vi "MAIN_STANDALONE.vi"() -> ()   [LabVIEW 2019]
uses:
  Type_defs/INPUT TEST.ctl
  Type_defs/OUTPUTS_TEST.ctl
  LVPROJ_CONFIG_ESTACION/Type_defs/Coordenadas_estacion.ctl
  LVPROJ_CREAR BANDEJAS/Type_defs/Data_Bandeja.ctl
  Type_defs/State_main.ctl
  LVPROJ_MOVIMIENTO_CABEZAL/LABVIEW_MOVIMIENTO/MOVIMIENTO CABEZAL/Typedefs/Comandos.ctl
  LVPROJ_MOVIMIENTO_CABEZAL/LABVIEW_MOVIMIENTO/MOVIMIENTO CABEZAL/Typedefs/Estados_arduino.ctl
  <vilib>/Instr/_visa.llb/VISA Configure Serial Port (Instr).vi
  <vilib>/Utility/error.llb/Error Cluster From Error Code.vi
  <vilib>/ErrorRing/Error Ring.xnode
  SHARED VI'S/SHARED VI'S.lvlib
panel:
  out "datos leídos por arduino":string
  out "CONEXION CON ARDUINO":bool
  out "read buffer 2":string
  out "read buffer":string
  out "trama datos enviada":string
  out "datos enviados = datos leídos?":bool
  out "Error Out":errorcluster
  in  "Error In":errorcluster
  in  "Tab Control":enum32{"PANEL USUARIO", "VER CONFIG ACTUAL"}(tab)
  in  "COMENZAR TEST":bool
  in  "EXIT":bool
  in  "DETENER TEST":bool
  in  "ENVIAR PARAMETROS DE TEST":bool
  in  "TEST ASICS INPUT":T1={"COORD. IN X"=0, "COORD IN Y"=0, "COORD OK X"=0, "COORD OK Y"=0, "COORD NOK X"=0, "COORD NOK Y"=0, "NºASICS A TESTEAR"=1, "SELECCIÓN DE TEST"=enum."TEST ASICS LST", "CUENTA ASICS"=0, "OPERADOR"="Javier Morales"}
  out "INDICADORES DE TEST":T2
  out "ESTADO FSM":T3
  out "Configuracion Estación":T4={"Coordenadas_estacion"={"Coord.Bandeja entrada"={"Coord. X0 entrada"=0, "Coord. Y0 entrada "=0, "Altura Z entrada"=0}, "Coord.Bandeja OK"={"Coord. X0 OK"=0, "Coord. Y0 OK"=0, "Altura Z OK"=0}, "Coord.Bandeja entrada FAIL"={"Coord. X0 FAIL"=0, "Coord. Y0 FAIL"=0, "Altura Z FAIL"=0}, "Coord. Socket"={"Coord. X socket"=0, "Coord. Y socket"=0, "Altura Z socket"=0}}, "Nombre Bandeja"="", "Datos bandeja"={"Nº de columnas "=0, "Nº de filas "=0, "largo"=0, "ancho"=0, "nombre"="nombre", "Paso X (en mm)"=0.0, "Paso Y (en mm)"=0.0, "DISTANCIA SUELO A CHIP  "=0.0, "Nº de celdas totales"=0, "Distancia chips bandejas contiguas"=0.0}}
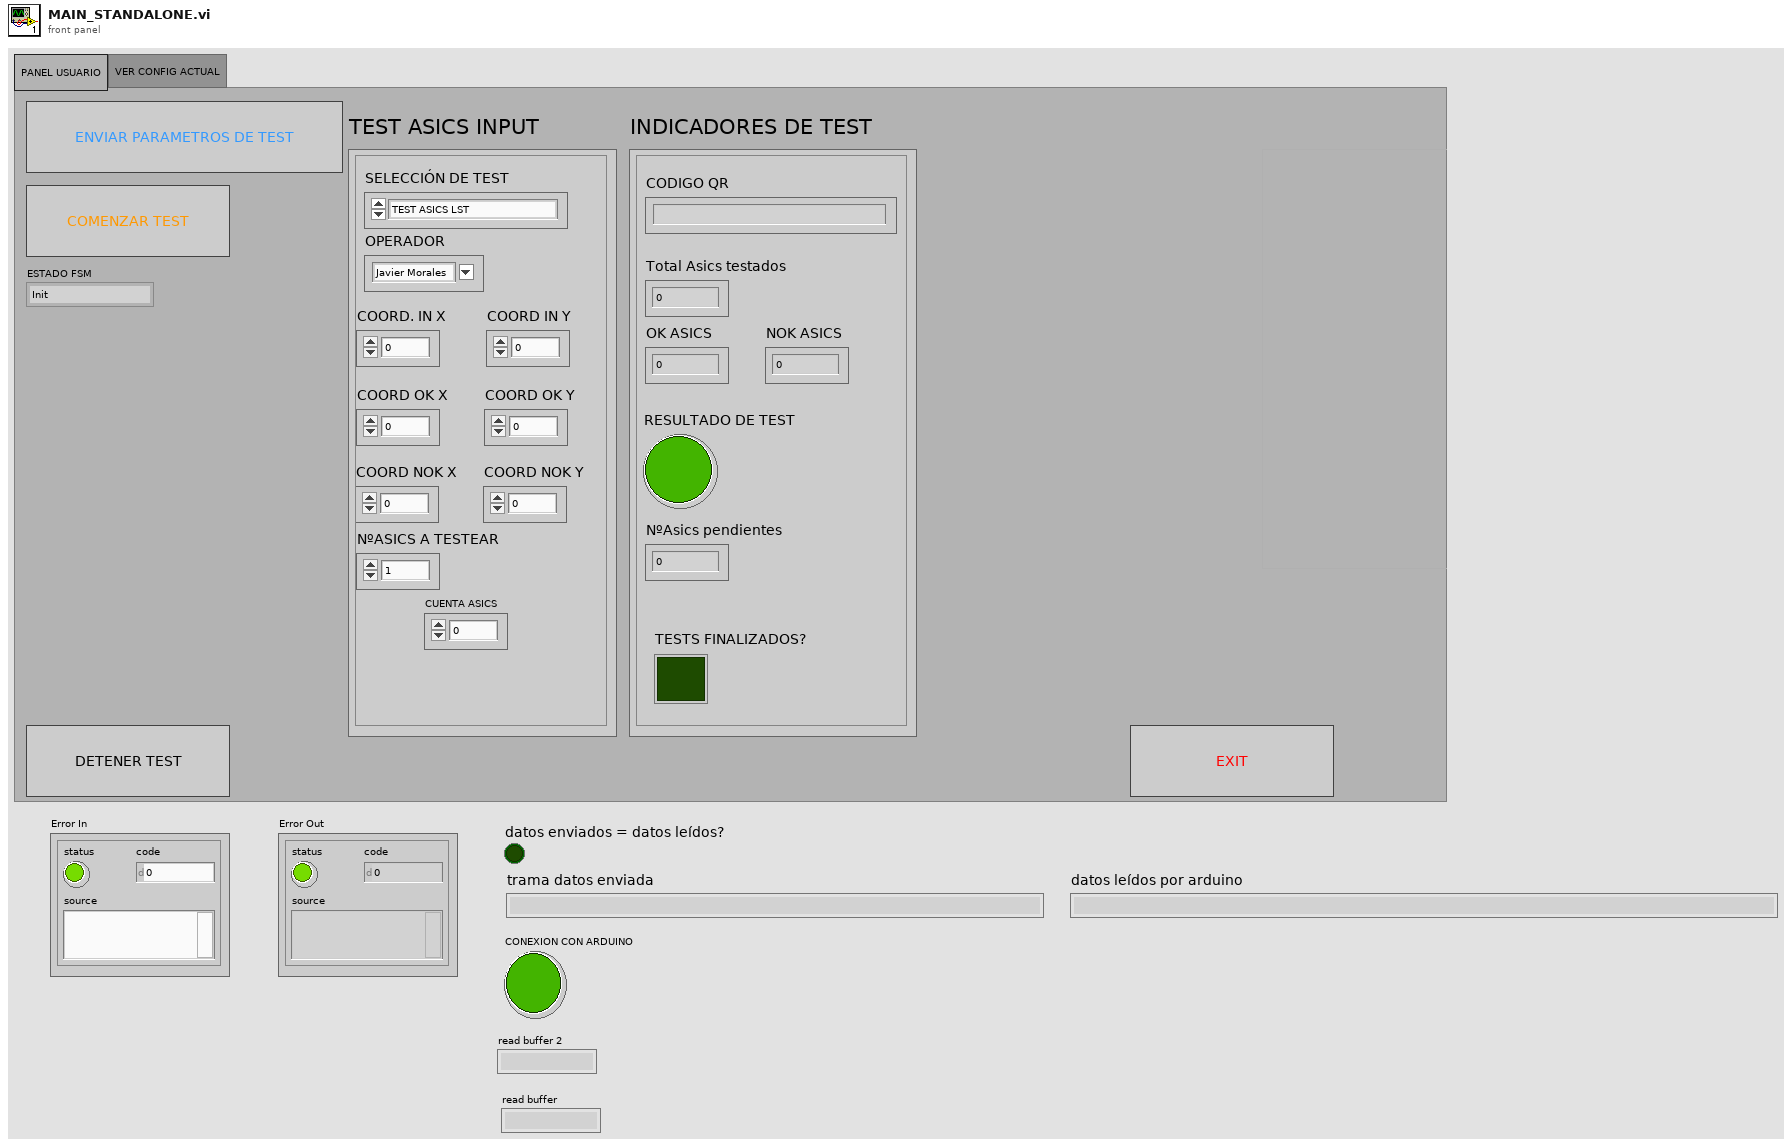
[diagram p1: front panel]
types:
  T1 = typedef "INPUT TEST.ctl" = cluster{"COORD. IN X":u16, "COORD IN Y":u16, "COORD OK X":u16, "COORD OK Y":u16, "COORD NOK X":u16, "COORD NOK Y":u16, "NºASICS A TESTEAR":u32, "SELECCIÓN DE TEST":enum16{"TEST ASICS LST"}, "CUENTA ASICS":u32, "OPERADOR":string}
  T2 = typedef "OUTPUTS_TEST.ctl" = cluster{"CODIGO QR":string, "OK ASICS":u32, "NOK ASICS":u32, "RESULTADO DE TEST":bool, "TESTS FINALIZADOS?":bool, "Total Asics testados":u32, "NºAsics pendientes":u32}
  T3 = typedef "State_main.ctl" = enum16{"Init", "Wait for Event", "Init refs", "Init com", "Config estacion", "Home", "Ping_Arduino", "Coge Asic", "Enviar_config_test", "Test_call", "Dejar Asic", "Leer QR", "Ejecutar Test", "Actualizar valores", "Enviar resultadoTest Arduino", "Final de test?", "Terminar", "Exit", "Error?"}
  T4 = typedef "Configuracion_estación.ctl" = cluster{"Coordenadas_estacion":T5, "Nombre Bandeja":string, "Datos bandeja":T6}
  T5 = typedef "Coordenadas_estacion.ctl" = cluster{"Coord.Bandeja entrada":cluster{"Coord. X0 entrada":u32, "Coord. Y0 entrada ":u32, "Altura Z entrada":u32}, "Coord.Bandeja OK":cluster{"Coord. X0 OK":u32, "Coord. Y0 OK":u32, "Altura Z OK":u32}, "Coord.Bandeja entrada FAIL":cluster{"Coord. X0 FAIL":u32, "Coord. Y0 FAIL":u32, "Altura Z FAIL":u32}, "Coord. Socket":cluster{"Coord. X socket":u32, "Coord. Y socket":u32, "Altura Z socket":u32}}
  T6 = typedef "Data_Bandeja.ctl" = cluster{"Nº de columnas ":u32, "Nº de filas ":u32, "largo":u32, "ancho":u32, "nombre":string, "Paso X (en mm)":dbl, "Paso Y (en mm)":dbl, "DISTANCIA SUELO A CHIP  ":dbl, "Nº de celdas totales":u16, "Distancia chips bandejas contiguas":dbl}
  T7 = typedef "Comandos.ctl" = enum16{"H", "FH", "FM", "FI", "FX", "FY", "FZ", "I", "OK"}
  T8 = typedef "Estados_arduino.ctl" = enum16{"2", "3", "4", "5", "6", "7", "9", "8"}
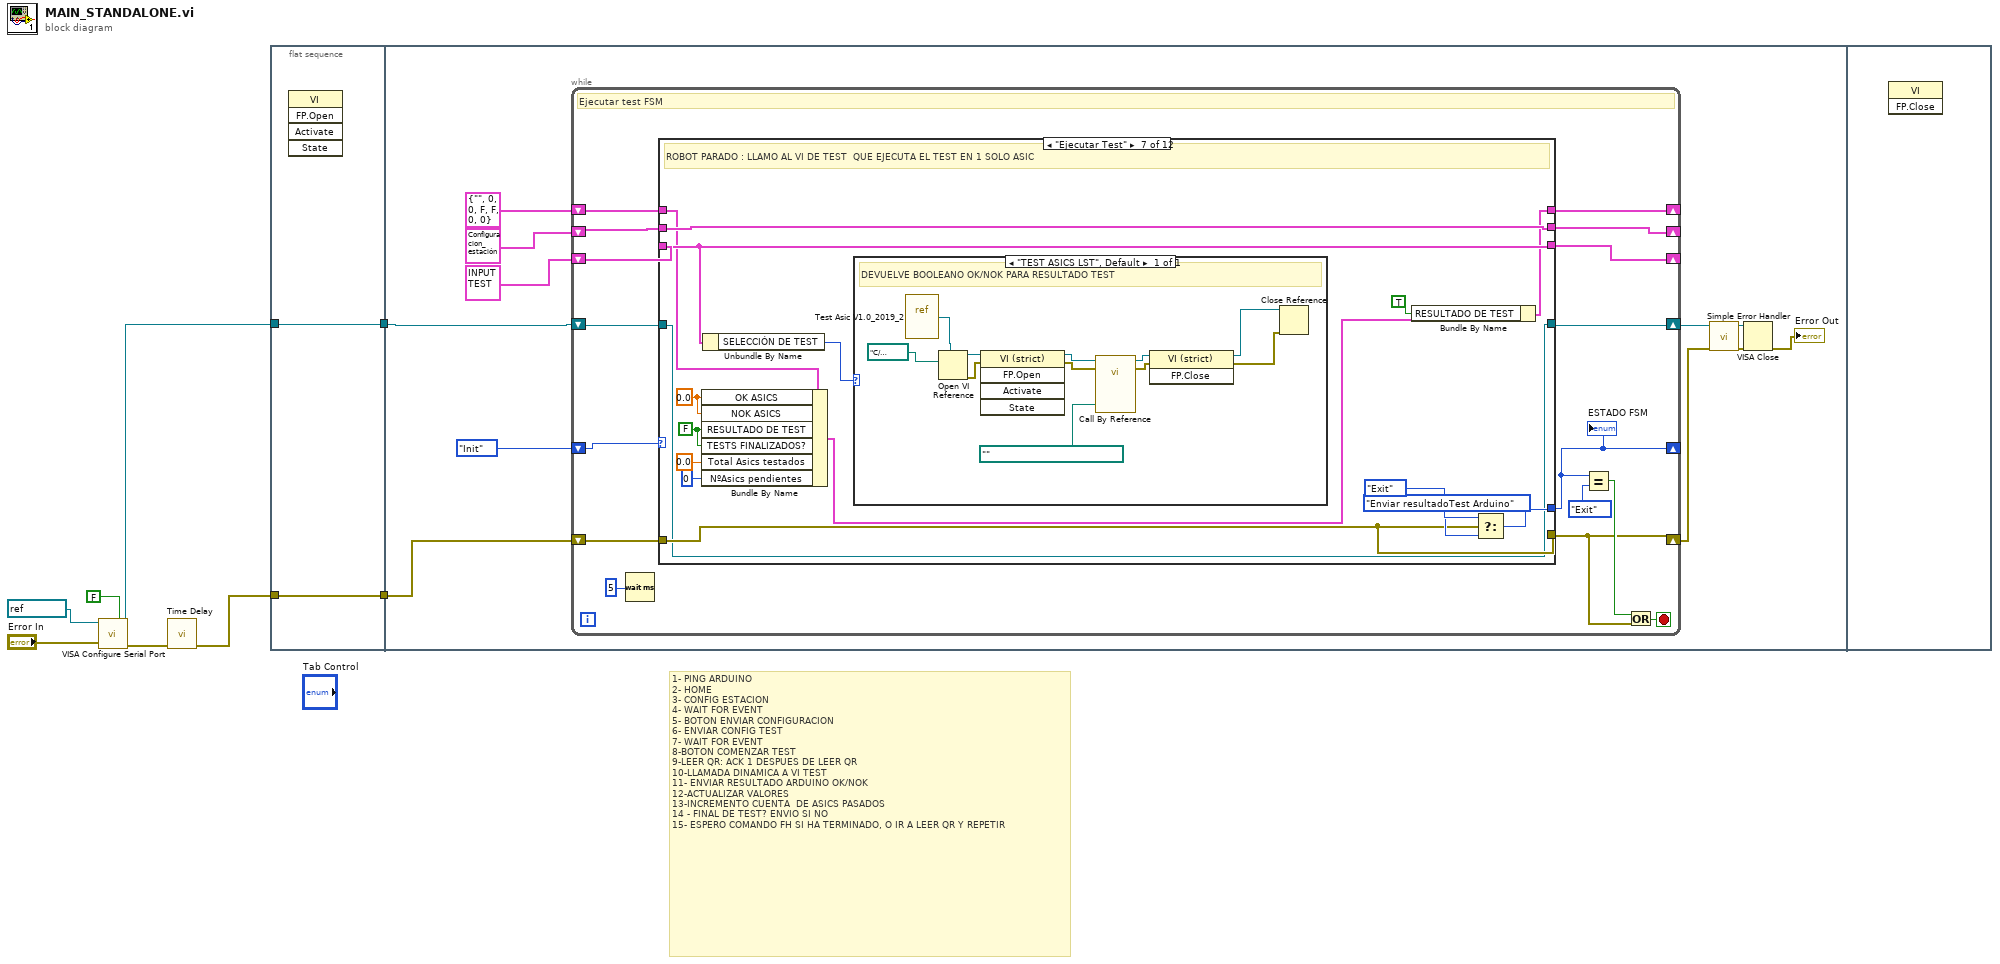
[diagram p0: block diagram]
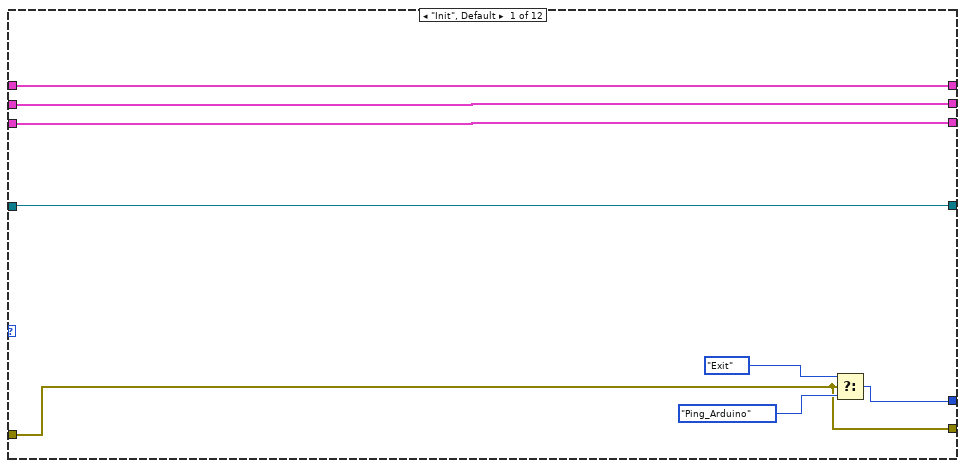
[diagram p2: hidden frame]
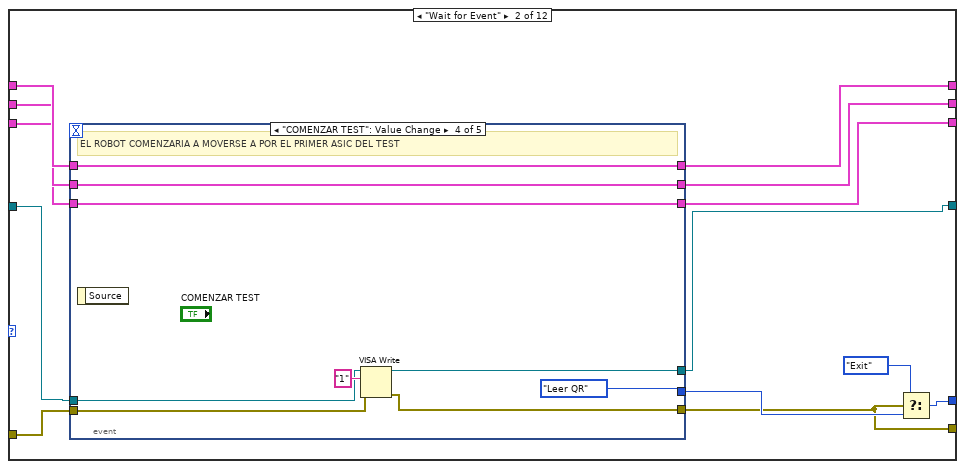
[diagram p3: hidden frame]
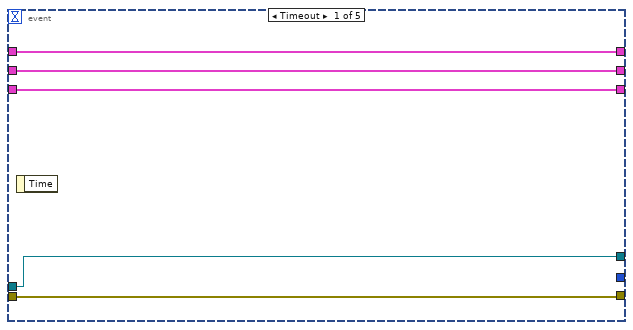
[diagram p4: hidden frame]
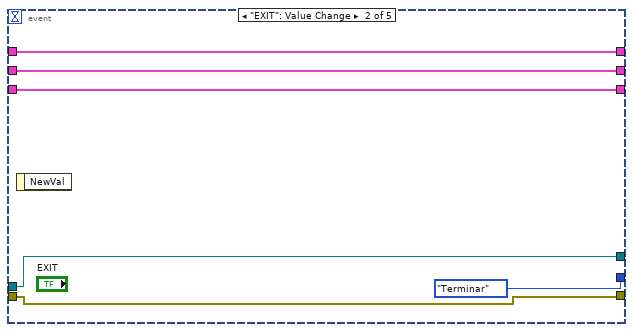
[diagram p5: hidden frame]
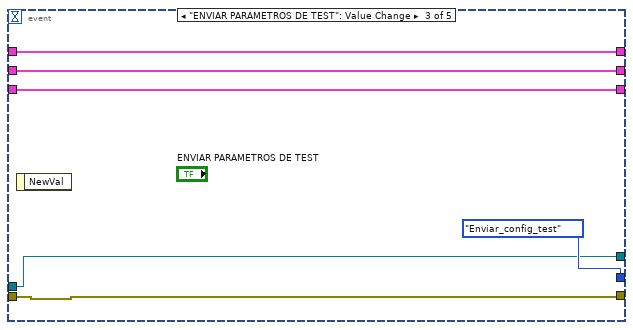
[diagram p6: hidden frame]
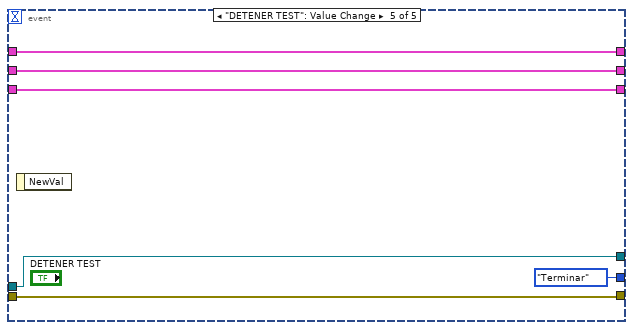
[diagram p7: hidden frame]
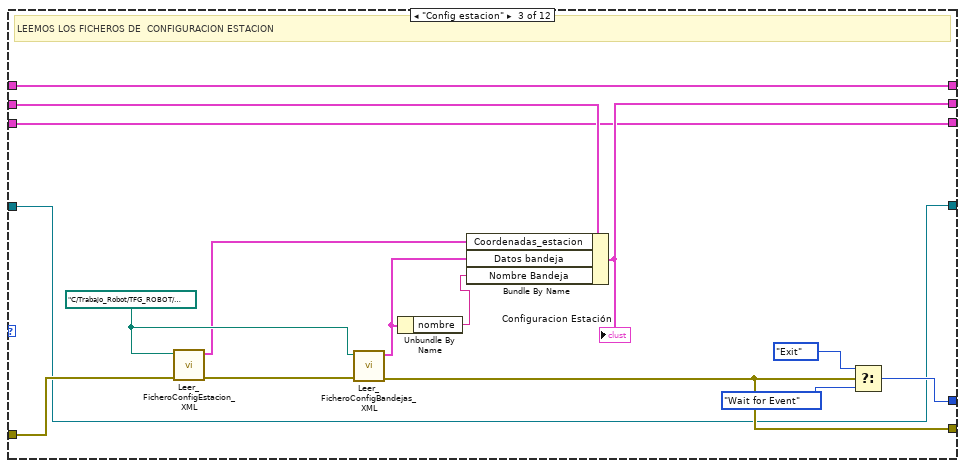
[diagram p8: hidden frame]
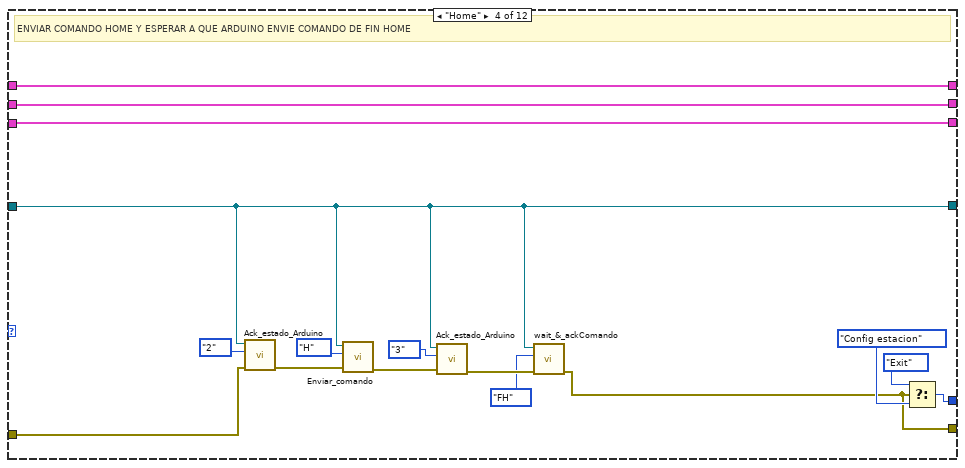
[diagram p9: hidden frame]
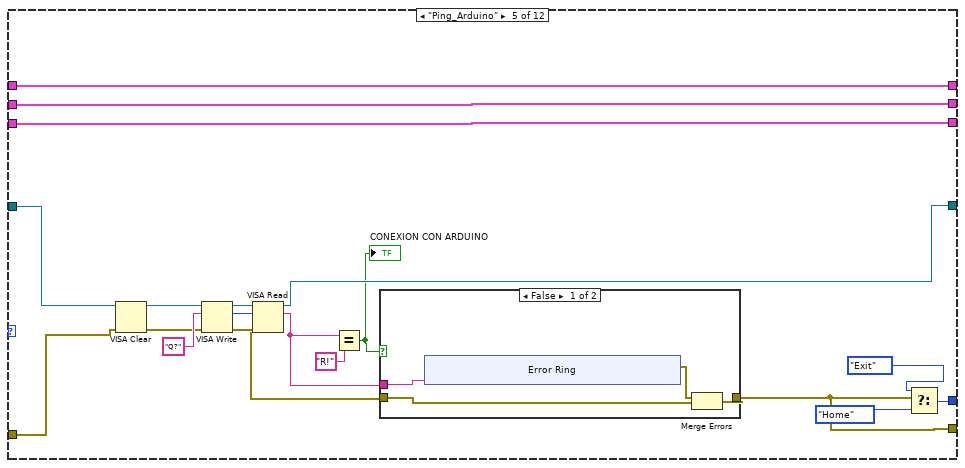
[diagram p10: hidden frame]
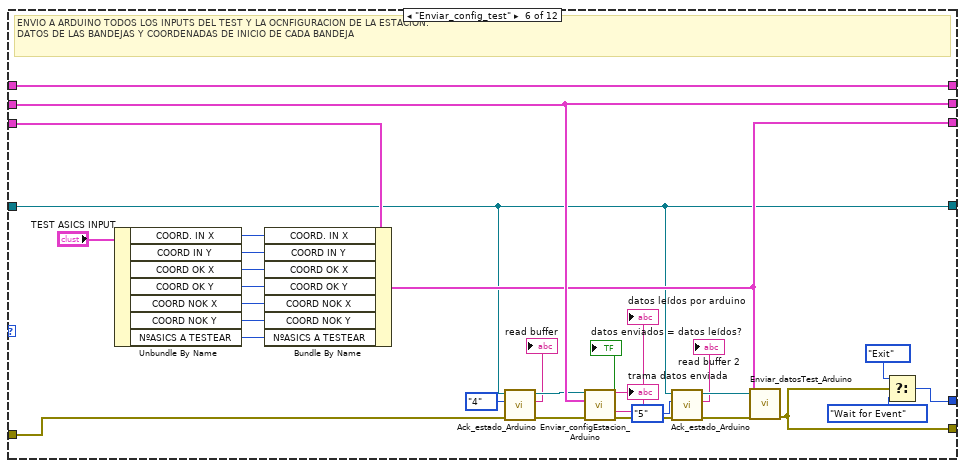
[diagram p12: hidden frame]
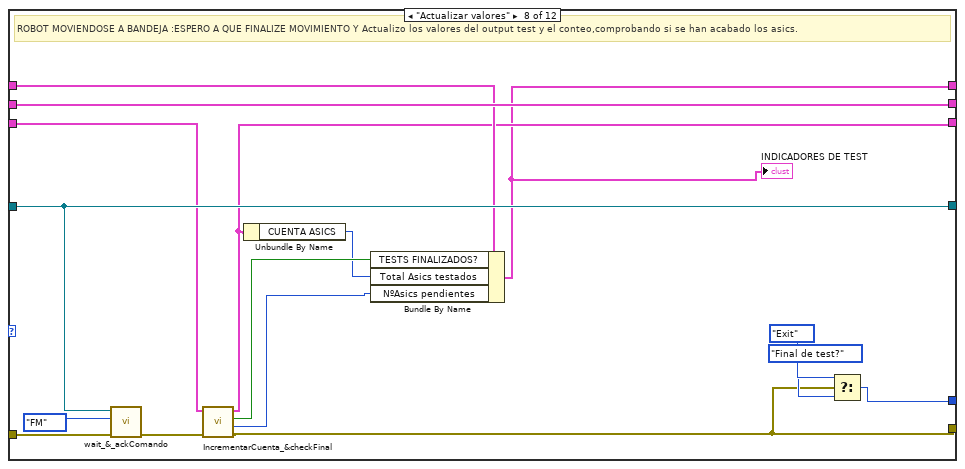
[diagram p13: hidden frame]
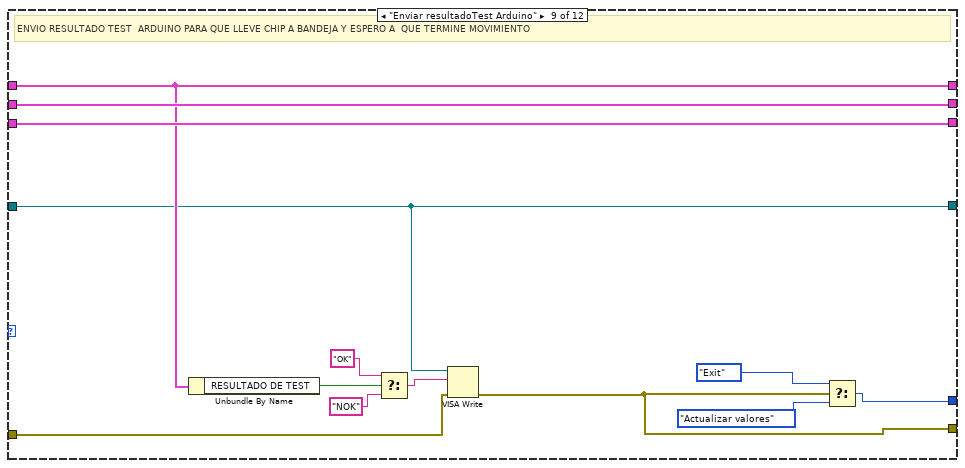
[diagram p14: hidden frame]
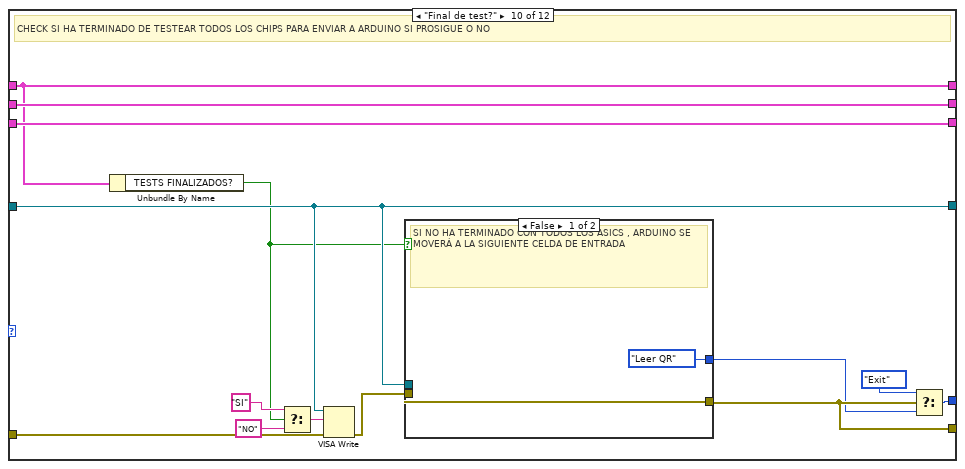
[diagram p15: hidden frame]
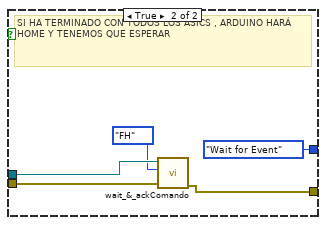
[diagram p16: hidden frame]
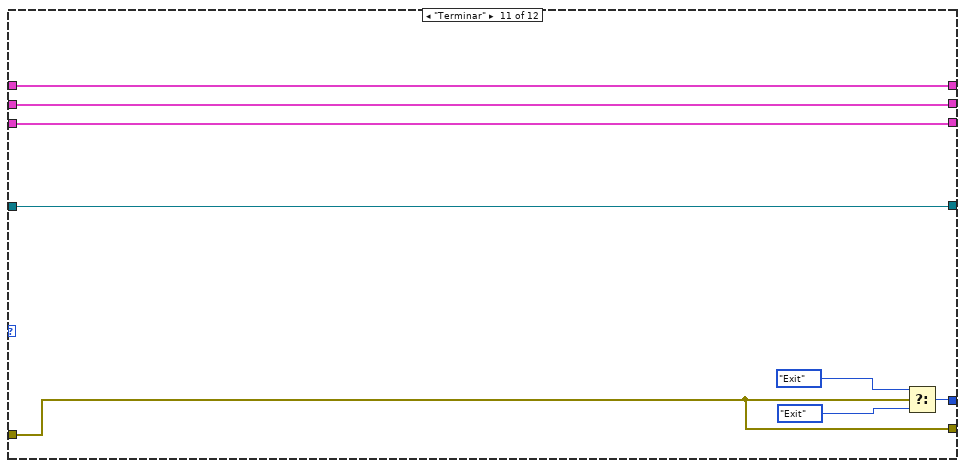
[diagram p17: hidden frame]
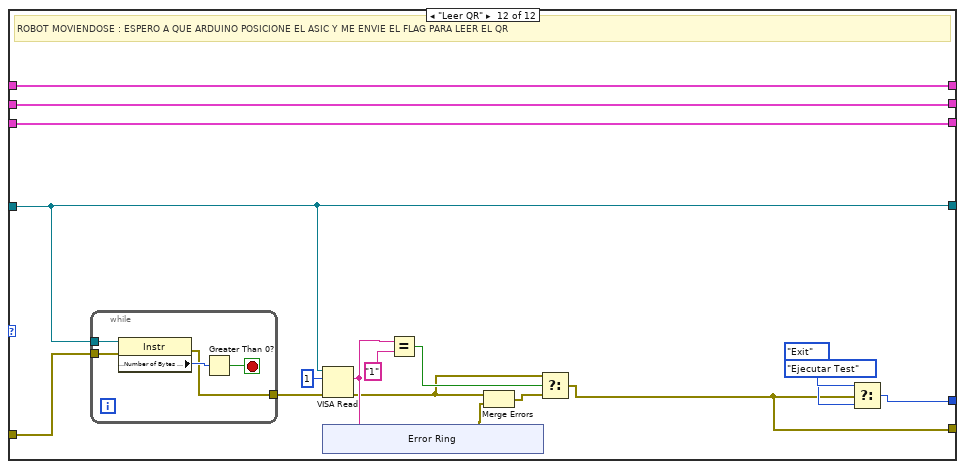
[diagram p18: hidden frame]
diagram:
  # "1- PING ARDUINO\n2- HOME\n3- CONFIG ESTACION\n4- WAIT FOR EVENT\n5- BOTON ENVIAR CONFIGURACION\n6- ENVIAR CONFIG TEST\n7- WAIT FOR EVENT\n8-BOTON COMENZAR TEST\n9-LEER QR: ACK 1 DESPUES DE LEER QR\n10-LLAMADA DINAMICA A VI TEST\n11- ENVIAR RESULTADO ARDUINO OK/NOK\n12-ACTUALIZAR VALORES\n13-INCREMENTO CUENTA  DE ASICS PASADOS\n14 - FINAL DE TEST? ENVIO SI NO\n15- ESPERO COMANDO FH SI HA TERMINADO, O IR A LEER QR Y REPETIR"
  n1 = call-poly "VISA Configure Serial Port"("VISA resource name"=refnum<visa-resource-name> "COM4", "Enable Termination\nChar (T)"=FALSE ("Enable Termination\nChar (T)"), "error in (no error)"="Error In") -> ("VISA resource name out"=w2:refnum<visa-resource-name>, "error out"=w5:errorcluster)  [unwired: 11 in]
  n2 = call "Time Delay"("error in (no error)"=w5) -> ("error out"=w4:errorcluster)  [unwired: 10 in]
  n3 = flat-sequence {
    tunnel: w4 -> [w10]
    tunnel: [w10] -> w3
    tunnel: w2 -> [w9]
    tunnel: [w9] -> w1
    tunnel: w3 -> [w17]
    tunnel: w1 -> [w16]
    frame #0 {
      n4 = invoke class="VI" method="FP.Open"() -> ()  [unwired: 5 in, 5 out]
    }
    frame #1 {
      n5 = while {
        shift-right: [w29] -> _
        shift-left: State_main."Init" ("States_main") -> [w36]
        shift-right: [w30] -> w13
        shift-left: w17 -> [w34]
        shift-right: [w22] -> _
        shift-left: T1 {"COORD. IN X"=0, "COORD IN Y"=0, "COORD OK X"=0, "COORD OK Y"=0, "COORD NOK X"=0, "COORD NOK Y"=0, "NºASICS A TESTEAR"=1, "SELECCIÓN DE TEST"=enum."TEST ASICS LST", "CUENTA ASICS"=0, "OPERADOR"="Javier Morales"} ("TEST ASICS INPUT") -> [w33]
        shift-right: [w24] -> _
        shift-left: T4 {"Coordenadas_estacion"={"Coord.Bandeja entrada"={"Coord. X0 entrada"=0, "Coord. Y0 entrada "=0, "Altura Z entrada"=0}, "Coord.Bandeja OK"={"Coord. X0 OK"=0, "Coord. Y0 OK"=0, "Altura Z OK"=0}, "Coord.Bandeja entrada FAIL"={"Coord. X0 FAIL"=0, "Coord. Y0 FAIL"=0, "Altura Z FAIL"=0}, "Coord. Socket"={"Coord. X socket"=0, "Coord. Y socket"=0, "Altura Z socket"=0}}, "Nombre Bandeja"="", "Datos bandeja"={"Nº de columnas "=0, "Nº de filas "=0, "largo"=0, "ancho"=0, "nombre"="nombre", "Paso X (en mm)"=0.0, "Paso Y (en mm)"=0.0, "DISTANCIA SUELO A CHIP  "=0.0, "Nº de celdas totales"=0, "Distancia chips bandejas contiguas"=0.0}} ("Configuracion Estación") -> [w28]
        shift-right: [w26] -> w11
        shift-left: w16 -> [w27]
        shift-right: [w23] -> _
        shift-left: T2 {"CODIGO QR"="", "OK ASICS"=0, "NOK ASICS"=0, "RESULTADO DE TEST"=FALSE, "TESTS FINALIZADOS?"=FALSE, "Total Asics testados"=0, "NºAsics pendientes"=0} -> [w25]
        stop <- w32 stop-if-true
        # "Ejecutar test FSM"
        n6 = Wait (ms)(milliseconds to wait=u32 5) -> ()  [unwired: 1 out]
        n7 = case shown="\"Ejecutar Test\"" w36 {
          tunnel: w34 -> [w37 w48 w101 w108 w124 w165 w194 w220 w227 w245 w261 w284]
          tunnel: w33 -> [w39 w50 w90 w115 w135 w179 w192 w218 w234 w249 w263 w278]
          tunnel: [w42 w56 w102 w118 w138 w180 w196 w223 w236 w251 w260 w281] -> w29
          tunnel: [w37 w47 w95 w107 w127 w168 w194 w216 w226 w243 w261 w268] -> w30
          tunnel: w28 -> [w40 w52 w93 w116 w136 w169 w193 w222 w235 w250 w264 w279]
          tunnel: w27 -> [w38 w46 w94 w105 w122 w160 w191 w221 w228 w242 w262 w275]
          tunnel: [w38 w45 w94 w105 w126 w160 w191 w221 w228 w242 w262 w275] -> w26
          tunnel: w25 -> [w41 w54 w91 w117 w137 w170 w184 w214 w233 w239 w265 w280]
          tunnel: [w40 w51 w92 w116 w136 w169 w193 w222 w235 w250 w264 w279] -> w24
          tunnel: [w41 w53 w91 w117 w137 w170 w189 w210 w233 w239 w265 w280] -> w23
          tunnel: [w39 w49 w90 w115 w135 w167 w192 w213 w234 w249 w263 w278] -> w22
          frame "Init", Default {
            n8 = Select(t=State_main."Exit" ("States_main"), s=w37, f=State_main."Ping_Arduino" ("States_main")) -> (s? t:f=w42:T3)
          }
          frame "Wait for Event" {
            n9 = event shown="[3] \"COMENZAR TEST\": Value Change" {
              selector: _ -> [_ _ _ _ _]
              dyn-events: _ -> [_ _ _ _ _]
              timeout: _ -> [_ _ _ _ _]
              tunnel: [_ State_main."Terminar" ("States_main") State_main."Enviar_config_test" ("States_main") State_main."Leer QR" ("States_main") State_main."Terminar" ("States_main")] -> w55
              tunnel: w54 -> [w62 w67 w73 w82 w89]
              tunnel: [w62 w67 w73 w82 w89] -> w53
              tunnel: w52 -> [w61 w66 w72 w81 w88]
              tunnel: [w61 w66 w72 w81 w88] -> w51
              tunnel: w50 -> [w60 w65 w71 w80 w87]
              tunnel: [w60 w65 w71 w80 w87] -> w49
              tunnel: w48 -> [w59 w64 w70 w76 w85]
              tunnel: [w59 w64 w70 w75 w85] -> w47
              tunnel: w46 -> [w58 w63 w69 w78 w84]
              tunnel: [w58 w63 w69 w77 w84] -> w45
              event Timeout {
                n10 = event-data() -> ()  [unwired: 1 in, 1 out]
              }
              event "EXIT": Value Change {
                n11 = event-data() -> ()  [unwired: 1 in, 1 out]
              }
              event "ENVIAR PARAMETROS DE TEST": Value Change {
                n12 = event-data() -> ()  [unwired: 1 in, 1 out]
              }
              event "COMENZAR TEST": Value Change {
                # "EL ROBOT COMENZARIA A MOVERSE A POR EL PRIMER ASIC DEL TEST"
                n13 = event-data() -> ()  [unwired: 1 in, 1 out]
                n14 = VISA Write(VISA resource name=w78, write buffer="1", error in (no error)=w76) -> (VISA resource name out=w77:refnum<visa-resource-name>, error out=w75:errorcluster)  [unwired: 1 out]
              }
              event "DETENER TEST": Value Change {
                n15 = event-data() -> ()  [unwired: 1 in, 1 out]
              }
            }
            n16 = Select(t=State_main."Exit" ("States_main"), s=w47, f=w55) -> (s? t:f=w56:T3)
          }
          frame "Config estacion" {
            w99 = path "C:/Trabajo_Robot/TFG_ROBOT/CONTROL_ROBOT/LABVIEW_ROBOT_MASTER" ("XML File Path")
            # "LEEMOS LOS FICHEROS DE  CONFIGURACION ESTACION"
            n17 = call "Leer_FicheroConfigEstacion_XML.vi"("error in (no error)"=w101, "XML File Path"=w99) -> ("error out"=w100:errorcluster, "Coordenadas_estacion"=w98:T5)  [unwired: 8 in]
            n18 = call "Leer_FicheroConfigBandejas_XML.vi"("error in (no error)"=w100, "XML File Path"=w99) -> ("error out"=w95:errorcluster, "Datos bandeja"=w97:T6)  [unwired: 8 in]
            n19 = Unbundle By Name(w97) -> ("nombre"=w96:string)
            n20 = Bundle By Name(cluster=w93, "Coordenadas_estacion"=w98, "Datos bandeja"=w97, "Nombre Bandeja"=w96) -> (w92:T4)
            "Configuracion Estación" <- w92
            n21 = Select(t=State_main."Exit" ("States_main"), s=w95, f=State_main."Wait for Event" ("States_main")) -> (s? t:f=w102:T3)
          }
          frame "Home" {
            # "ENVIAR COMANDO HOME Y ESPERAR A QUE ARDUINO ENVIE COMANDO DE FIN HOME"
            n22 = call "Ack_estado_Arduino.vi"("error in (no error)"=w108, "Enum"=Estados_arduino."2", "VISA resource name"=w105) -> ("error out"=w114:errorcluster)  [unwired: 6 in, 2 out]
            n23 = call "Enviar_comando.vi"("error in (no error)"=w114, "Enum"=Comandos."H", "VISA resource name"=w105) -> ("error out"=w109:errorcluster)  [unwired: 6 in, 2 out]
            n24 = call "Ack_estado_Arduino.vi"("error in (no error)"=w109, "Enum"=Estados_arduino."3", "VISA resource name"=w105) -> ("error out"=w110:errorcluster)  [unwired: 6 in, 2 out]
            n25 = call "wait_&_ackComando.vi"("error in (no error)"=w110, 10:Comandos."FH", "VISA Refnum in"=w105) -> ("error out"=w107:errorcluster)  [unwired: 7 in, 1 out]
            n26 = Select(t=State_main."Exit" ("States_main"), s=w107, f=State_main."Config estacion" ("States_main")) -> (s? t:f=w118:T3)
          }
          frame "Ping_Arduino" {
            n27 = VISA Clear(VISA resource name=w122, error in (no error)=w124) -> (VISA resource name out=w121:refnum<visa-resource-name>, error out=w123:errorcluster)
            n28 = VISA Write(VISA resource name=w121, write buffer="Q?", error in (no error)=w123) -> (VISA resource name out=w128:refnum<visa-resource-name>, return count=w133:u32, error out=w132:errorcluster)
            n29 = VISA Read(VISA resource name=w128, byte count=w133, error in (no error)=w132) -> (VISA resource name out=w126:refnum<visa-resource-name>, read buffer=w130:string, error out=w129:errorcluster)  [unwired: 1 out]
            n30 = Equal?(x=w130, y="R!") -> (x = y?=w125:bool)
            "CONEXION CON ARDUINO" <- w125
            n31 = case shown="False" w125 {
              tunnel: w130 -> [w144 _]
              tunnel: w129 -> [w142 w152]
              tunnel: [w141 w152] -> w127
              frame False {
                n32 = xnode "Error Ring"("parameter 0"=w144) -> ("error out"=w143:errorcluster)
                n33 = Merge Errors(w143, w142) -> (w141:errorcluster)
              }
              frame True {
              }
            }
            n34 = Select(t=State_main."Exit" ("States_main"), s=w127, f=State_main."Home" ("States_main")) -> (s? t:f=w138:T3)
          }
          frame "Enviar_config_test" {
            # "ENVIO A ARDUINO TODOS LOS INPUTS DEL TEST Y LA OCNFIGURACION DE LA ESTACIÓN:\nDATOS DE LAS BANDEJAS Y COORDENADAS DE INICIO DE CADA BANDEJA"
            n35 = Unbundle By Name("TEST ASICS INPUT") -> ("COORD. IN X"=w177:u16, "COORD IN Y"=w176:u16, "COORD OK X"=w175:u16, "COORD OK Y"=w174:u16, "COORD NOK X"=w173:u16, "COORD NOK Y"=w172:u16, "NºASICS A TESTEAR"=w171:u32)
            n36 = Bundle By Name(cluster=w179, "COORD. IN X"=w177, "COORD IN Y"=w176, "COORD OK X"=w175, "COORD OK Y"=w174, "COORD NOK X"=w173, "COORD NOK Y"=w172, "NºASICS A TESTEAR"=w171) -> (w167:T1)
            n37 = call "Ack_estado_Arduino.vi"("error in (no error)"=w165, "Enum"=Estados_arduino."4", "VISA resource name"=w160) -> ("error out"=w164:errorcluster, "read buffer"=→"read buffer":string, "VISA resource name out"=w161:refnum<visa-resource-name>)  [unwired: 6 in]
            n38 = call "Enviar_configEstacion_Arduino.vi"("VISA resource name"=w161, "Configuracion Estación"=w169, "error in (no error)"=w164) -> ("trama datos enviada"=→"trama datos enviada":string, "datos enviados = datos leídos?"=→"datos enviados = datos leídos?":bool, "datos leídos"=→"datos leídos por arduino":string, "error IO"=w163:errorcluster)  [unwired: 9 in]
            n39 = call "Ack_estado_Arduino.vi"("error in (no error)"=w163, "Enum"=Estados_arduino."5", "VISA resource name"=w160) -> ("error out"=w162:errorcluster, "read buffer"=→"read buffer 2":string, "VISA resource name out"=w159:refnum<visa-resource-name>)  [unwired: 6 in]
            n40 = call "Enviar_datosTest_Arduino.vi"("error in (no error)"=w162, "TEST ASICS INPUT"=w167, "VISA resource name"=w159) -> ("error IO"=w168:errorcluster)  [unwired: 8 in]
            n41 = Select(t=State_main."Exit" ("States_main"), s=w168, f=State_main."Wait for Event" ("States_main")) -> (s? t:f=w180:T3)
          }
          frame "Ejecutar Test" {
            w185 = FALSE ("RESULTADO DE TEST")
            w188 = 0.0 ("OK ASICS")
            # "ROBOT PARADO : LLAMO AL VI DE TEST  QUE EJECUTA EL TEST EN 1 SOLO ASIC"
            n42 = Bundle By Name(cluster=w184, "OK ASICS"=w188, "NOK ASICS"=w188, "RESULTADO DE TEST"=w185, "TESTS FINALIZADOS?"=w185, "Total Asics testados"=0.0, "NºAsics pendientes"=u32 0) -> (w183:T2)
            n43 = Unbundle By Name(w192) -> ("SELECCIÓN DE TEST"=w195:enum16{"TEST ASICS LST"})
            n44 = case shown="\"TEST ASICS LST\", Default" w195 {
              frame "TEST ASICS LST", Default {
                # "DEVUELVE BOOLEANO OK/NOK PARA RESULTADO TEST"
                n45 = vi-ref "Test Asic V1.0_2019_2.vi"() -> (w208:refnum<vi>)
                n46 = Open VI Reference(type specifier VI Refnum (for type only)=w208, vi path=path "C:/Trabajo_Robot/Test Asic Javi_2021/Test Asic V1.0_2019_2.vi") -> (vi reference=w207:refnum<vi>, error out=w205:errorcluster)  [unwired: 4 in]
                n47 = invoke class="VI (strict)" method="FP.Open"(reference=w207, error in=w205) -> (reference out=w206:refnum<vi>, error out=w204:errorcluster)  [unwired: 3 in, 3 out]
                n48 = call-by-ref "?"(reference=w206, error in=w204, "Config File"=path "") -> (reference out=w203:refnum<vi>, error out=w202:errorcluster)  [unwired: 4 in, 1 out]
                n49 = invoke class="VI (strict)" method="FP.Close"(reference=w203, error in=w202) -> (reference out=w201:refnum<vi>, error out=w200:errorcluster)  [unwired: 1 in, 1 out]
                n50 = Close Reference(reference=w201, error in (no error)=w200) -> ()  [unwired: 1 out]
              }
            }
            n51 = Bundle By Name(cluster=w183, "RESULTADO DE TEST"=TRUE) -> (w189:T2)
            n52 = Select(t=State_main."Exit" ("States_main"), s=w194, f=State_main."Enviar resultadoTest Arduino" ("States_main")) -> (s? t:f=w196:T3)
          }
          frame "Actualizar valores" {
            # "ROBOT MOVIENDOSE A BANDEJA :ESPERO A QUE FINALIZE MOVIMIENTO Y Actualizo los valores del output test y el conteo,comprobando si se han acabado los asics."
            n53 = call "wait_&_ackComando.vi"("error in (no error)"=w220, 10:Comandos."FM", "VISA Refnum in"=w221) -> ("error out"=w217:errorcluster)  [unwired: 7 in, 1 out]
            n54 = call "IncrementarCuenta_&checkFinal.vi"("error in (no error)"=w217, "TEST ASICS INPUT in"=w218) -> ("error out"=w216:errorcluster, "Asics pendientes"=w211:u32, "FINAL ASICS??"=w215:bool, "TEST ASICS INPUT out"=w213:T1)  [unwired: 6 in]
            n55 = Unbundle By Name(w213) -> ("CUENTA ASICS"=w212:u32)
            n56 = Bundle By Name(cluster=w214, "TESTS FINALIZADOS?"=w215, "Total Asics testados"=w212, "NºAsics pendientes"=w211) -> (w210:T2)
            "INDICADORES DE TEST" <- w210
            n57 = Select(t=State_main."Exit" ("States_main"), s=w216, f=State_main."Final de test?" ("States_main")) -> (s? t:f=w223:T3)
          }
          frame "Enviar resultadoTest Arduino" {
            # "ENVIO RESULTADO TEST  ARDUINO PARA QUE LLEVE CHIP A BANDEJA Y ESPERO A  QUE TERMINE MOVIMIENTO"
            n58 = Unbundle By Name(w233) -> ("RESULTADO DE TEST"=w232:bool)
            n59 = Select(t="OK", s=w232, f="NOK") -> (s? t:f=w229:string)
            n60 = VISA Write(VISA resource name=w228, write buffer=w229, error in (no error)=w227) -> (error out=w226:errorcluster)  [unwired: 2 out]
            n61 = Select(t=State_main."Exit" ("States_main"), s=w226, f=State_main."Actualizar valores" ("States_main")) -> (s? t:f=w236:T3)
          }
          frame "Final de test?" {
            # "CHECK SI HA TERMINADO DE TESTEAR TODOS LOS CHIPS PARA ENVIAR A ARDUINO SI PROSIGUE O NO"
            n62 = Unbundle By Name(w239) -> ("TESTS FINALIZADOS?"=w240:bool)
            n63 = Select(t="SI", s=w240, f="NO") -> (s? t:f=w246:string)
            n64 = VISA Write(VISA resource name=w242, write buffer=w246, error in (no error)=w245) -> (error out=w244:errorcluster)  [unwired: 2 out]
            n65 = case shown="False" w240 {
              tunnel: w244 -> [w254 w257]
              tunnel: [w254 w255] -> w243
              tunnel: w242 -> [_ w258]
              tunnel: [State_main."Leer QR" ("States_main") State_main."Wait for Event" ("States_main")] -> w241
              frame False {
                # "SI NO HA TERMINADO CON TODOS LOS ASICS , ARDUINO SE MOVERÁ A LA SIGUIENTE CELDA DE ENTRADA"
              }
              frame True {
                # "SI HA TERMINADO CON TODOS LOS ASICS , ARDUINO HARÁ HOME Y TENEMOS QUE ESPERAR"
                n66 = call "wait_&_ackComando.vi"("error in (no error)"=w257, 10:Comandos."FH", "VISA Refnum in"=w258) -> ("error out"=w255:errorcluster)  [unwired: 7 in, 1 out]
              }
            }
            n67 = Select(t=State_main."Exit" ("States_main"), s=w243, f=w241) -> (s? t:f=w251:T3)
          }
          frame "Terminar" {
            n68 = Select(t=State_main."Exit" ("States_main"), s=w261, f=State_main."Exit" ("States_main")) -> (s? t:f=w260:T3)
          }
          frame "Leer QR" {
            # "ROBOT MOVIENDOSE : ESPERO A QUE ARDUINO POSICIONE EL ASIC Y ME ENVIE EL FLAG PARA LEER EL QR"
            n69 = while {
              tunnel: w275 -> [w296]
              tunnel: w284 -> [w293]
              tunnel: [w292] -> w277
              stop <- w294 stop-if-true
              n70 = property class="Instr"(reference=w296, error in=w293) -> (error out=w292:errorcluster, "Serial Settings:Number of Bytes at Serial Port"=w295:u32)  [unwired: 1 out]
              n71 = Greater Than 0?(x=w295) -> (x > 0?=w294:bool)
            }
            n72 = VISA Read(VISA resource name=w275, byte count=u32 1, error in (no error)=w277) -> (read buffer=w272:string, error out=w269:errorcluster)  [unwired: 2 out]
            n73 = xnode "Error Ring"("parameter 0"=w272) -> ("error out"=w271:errorcluster)
            n74 = Equal?(x=w272, y="1") -> (x = y?=w273:bool)
            n75 = Merge Errors(w269, w271) -> (w270:errorcluster)
            n76 = Select(t=w269, s=w273, f=w270) -> (s? t:f=w268:errorcluster)
            n77 = Select(t=State_main."Exit" ("States_main"), s=w268, f=State_main."Ejecutar Test" ("States_main")) -> (s? t:f=w281:T3)
          }
        }
        "ESTADO FSM" <- w29
        n78 = Equal?(x=w29, y=State_main."Exit") -> (x = y?=w35:bool)
        n79 = Or(x=w35, y=w30) -> (x .or. y?=w32:bool)
      }
      n80 = call <vilib>:"Simple Error Handler.vi"("error in (no error)"=w13) -> ("error out"=w12:errorcluster)  [unwired: 4 in, 4 out]
      n81 = VISA Close(VISA resource name=w11, error in (no error)=w12) -> (error out=→"Error Out":errorcluster)
    }
    frame #2 {
      n82 = invoke class="VI" method="FP.Close"() -> ()  [unwired: 3 in, 3 out]
    }
  }
